vi "time.vi"(1 "in":string="10:25:36") -> (0 "out":string)   [LabVIEW 2018]
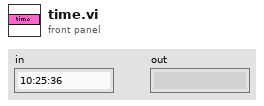
[diagram p1: front panel]
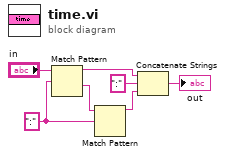
[diagram p0: block diagram]
diagram:
  w7 = ":"
  n1 = Match Pattern(string="in", regular expression=w7) -> (before substring=w4:string, after substring=w6:string)  [unwired: 1 in, 2 out]
  n2 = Match Pattern(string=w6, regular expression=w7) -> (before substring=w2:string)  [unwired: 1 in, 3 out]
  n3 = Concatenate Strings(w4, ":" ("string"), w2) -> (→"out":string)
